vi "saveImages.vi"   [LabVIEW 2012]
uses:
  GlobalBaslerCamera.vi
  <vilib>/Utility/file.llb/Write To Spreadsheet File (I64).vi
  Cpp Libraries/CatWalkLabviewDLL/labview code/OpenCvGlobals.vi
types:
  T1 = typedef "IMAQ Image.ctl" = refnum<image>
  T2 = typedef "Semaphore RefNum" = refnum<k1>
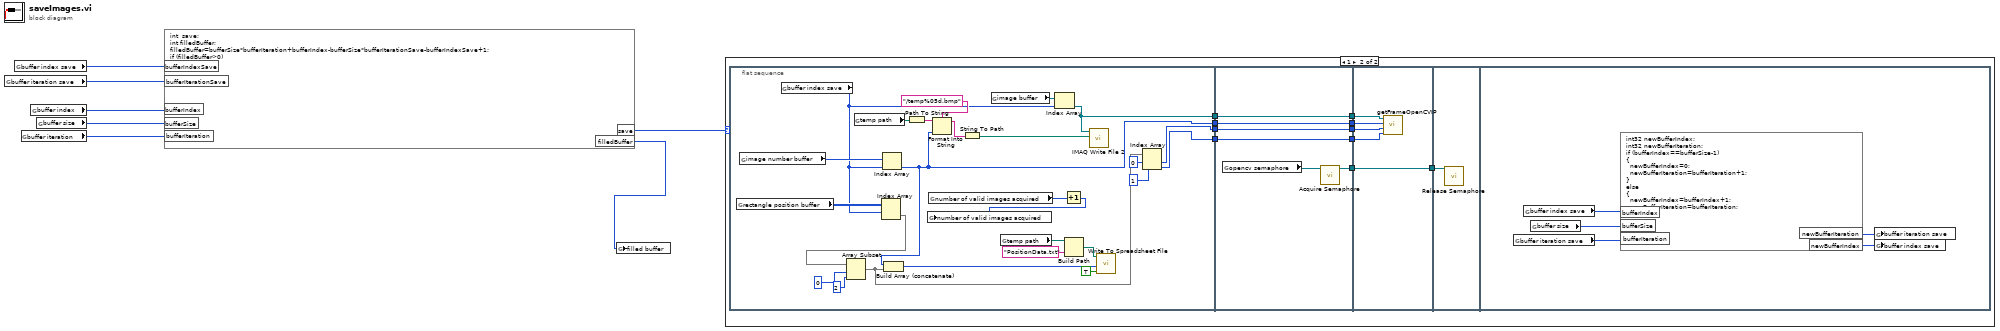
[diagram p0: block diagram]
diagram:
  n1 = global read "GlobalBaslerCamera.vi" "buffer iteration save"() -> (w3:i32)
  n2 = global read "GlobalBaslerCamera.vi" "buffer index save"() -> (w4:i32)
  n3 = global read "GlobalBaslerCamera.vi" "buffer iteration"() -> (w5:i32)
  n4 = global read "GlobalBaslerCamera.vi" "buffer index"() -> (w6:i32)
  n5 = global read "GlobalBaslerCamera.vi" "buffer size"() -> (w7:i32)
  n6 = formula code="int  save;\nint filledBuffer;\nfilledBuffer=bufferSize*bufferIteration+bufferIndex-bufferSize*bufferIterationSave-bufferIndexSave+1;\nif (filledBuffer>0)\nsave=1;\nelse\nsave=0;"("bufferIndex"=w6, "bufferSize"=w7, "bufferIteration"=w5, "bufferIndexSave"=w4, "bufferIterationSave"=w3) -> ("save"=w2:i32, "filledBuffer"=w1:i32)
  n7 = global write "GlobalBaslerCamera.vi" "filled buffer"(w1) -> ()
  n8 = case shown="1" w2 {
    frame 0, Default {
    }
    frame 1 {
      n9 = flat-sequence {
        tunnel: [w21] -> w17
        tunnel: [w20] -> w15
        tunnel: [w19] -> w13
        tunnel: [w18] -> w11
        tunnel: w17 -> [w49]
        tunnel: [w49] -> w16
        tunnel: w15 -> [w48]
        tunnel: [w48] -> w14
        tunnel: w13 -> [w47]
        tunnel: [w47] -> w12
        tunnel: w11 -> [w46]
        tunnel: [w46] -> w10
        tunnel: [w44] -> w8
        tunnel: w16 -> [w54]
        tunnel: w14 -> [w53]
        tunnel: w12 -> [w52]
        tunnel: w10 -> [w51]
        tunnel: [w50] -> w9
        tunnel: w8 -> [w50]
        tunnel: w9 -> [w55]
        frame #0 {
          n10 = global read "GlobalBaslerCamera.vi" "rectangle position buffer"() -> (w29:u16[][])
          n11 = global read "GlobalBaslerCamera.vi" "image number buffer"() -> (w37:u16[])
          n12 = global read "GlobalBaslerCamera.vi" "buffer index save"() -> (w28:i32)
          n13 = global read "GlobalBaslerCamera.vi" "temp path"() -> (w40:path)
          n14 = Index Array(array=w29, index (row)=w28) -> (element=w27:u16[])  [unwired: 1 in]
          n15 = Array Subset(array=w27, index=0, length=2) -> (w24:u16[])
          n16 = Index Array(array=w37, index=w28) -> (element=w20:u16)
          n17 = Build Array (concatenate)(w20, w24) -> (w34:u16[])
          n18 = Path To String(path=w40) -> (string=w41:string)
          n19 = global read "GlobalBaslerCamera.vi" "number of valid images acquired"() -> (w26:i32)
          n20 = Format Into String(format string="/temp%05d.bmp", initial string=w41, w20) -> (resulting string=w43:string)  [unwired: 1 in, 1 out]
          n21 = String To Path(string=w43) -> (path=w38:path)
          n22 = global read "GlobalBaslerCamera.vi" "image buffer"() -> (w39:T1[])
          n23 = global read "GlobalBaslerCamera.vi" "temp path"() -> (w32:path)
          n24 = Index Array(array=w39, index=w28) -> (element=w21:T1)
          n25 = Increment(x=w26) -> (x+1=w25:i32)
          n26 = global write "GlobalBaslerCamera.vi" "number of valid images acquired"(w25) -> ()
          n27 = Build Path(base path=w32, name or relative path="PositionData.txt") -> (appended path=w30:path)
          n28 = call-poly "IMAQ Write File 2"("File Path"=w38, "Image"=w21) -> ()  [unwired: 8 in, 2 out]
          n29 = call-poly <vilib>:"Write To Spreadsheet File.vi"("append to file? (new file:F)"=TRUE, "1D data"=w34, "file path (dialog if empty)"=w30) -> ()  [unwired: 5 in, 1 out]
          n30 = Index Array(array=w24, index #1=0 ("index"), index #2=1 ("index")) -> (element #1=w19:u16, element #2=w18:u16)
        }
        frame #1 {
          n31 = global read "OpenCvGlobals.vi" "opencv semaphore"() -> (w45:T2)
          n32 = call <vilib>:"Acquire Semaphore.vi"("semaphore"=w45) -> ("semaphore out"=w44:T2)  [unwired: 4 in, 2 out]
        }
        frame #2 {
          n33 = call "getFrameOpenCVIP.vi"("cropY"=w51, "cropX"=w52, "frameNumber"=w53, "Image"=w54) -> ()  [unwired: 1 out]
        }
        frame #3 {
          n34 = call <vilib>:"Release Semaphore.vi"("semaphore"=w55) -> ()  [unwired: 5 in, 2 out]
        }
        frame #4 {
          n35 = global read "GlobalBaslerCamera.vi" "buffer iteration save"() -> (w59:i32)
          n36 = global read "GlobalBaslerCamera.vi" "buffer index save"() -> (w58:i32)
          n37 = global read "GlobalBaslerCamera.vi" "buffer size"() -> (w60:i32)
          n38 = formula code="int32 newBufferIndex;\nint32 newBufferIteration;\nif (bufferIndex==bufferSize-1)\n{\n  newBufferIndex=0;\n  newBufferIteration=bufferIteration+1;\n}\nelse\n{\n  newBufferIndex=bufferIndex+1;\n  newBufferIteration=bufferIteration;\n}"("bufferIndex"=w58, "bufferSize"=w60, "bufferIteration"=w59) -> ("newBufferIndex"=w56:i32, "newBufferIteration"=w57:i32)
          n39 = global write "GlobalBaslerCamera.vi" "buffer iteration save"(w57) -> ()
          n40 = global write "GlobalBaslerCamera.vi" "buffer index save"(w56) -> ()
        }
      }
    }
  }
